vi "dataCube.vi"(10 "Enum":enum16{"clear", "read", "write"}(ring)=enum."write", 11 "imageCube":i32[][][](array[numeric])) -> (1 "imageCubeBkgSubstractedRefDivided":i32[][][](array[numeric]), 2 "imageCubeBkgSubstracted":i32[][][](array[numeric]), 3 "imageCubeOut":i32[][][](array[numeric]))   [LabVIEW 2016]
uses:
  imageSettings.vi
panel:
  out "ref":i32[][](graph)
  out "bkg":i32[][](graph)
  out "raw":i32[][](graph)
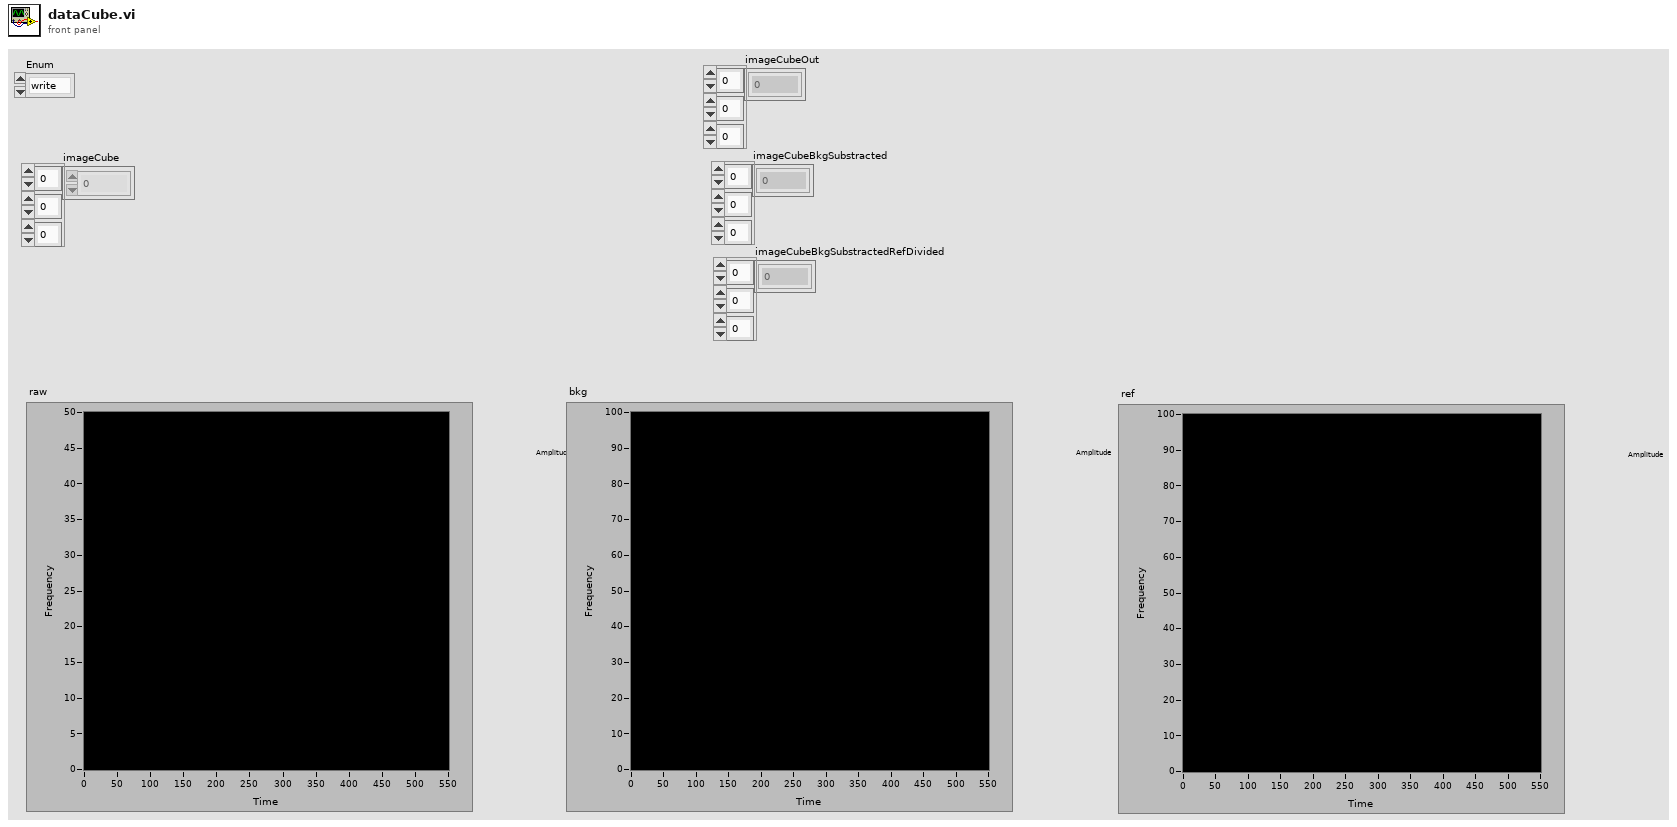
[diagram p1: front panel]
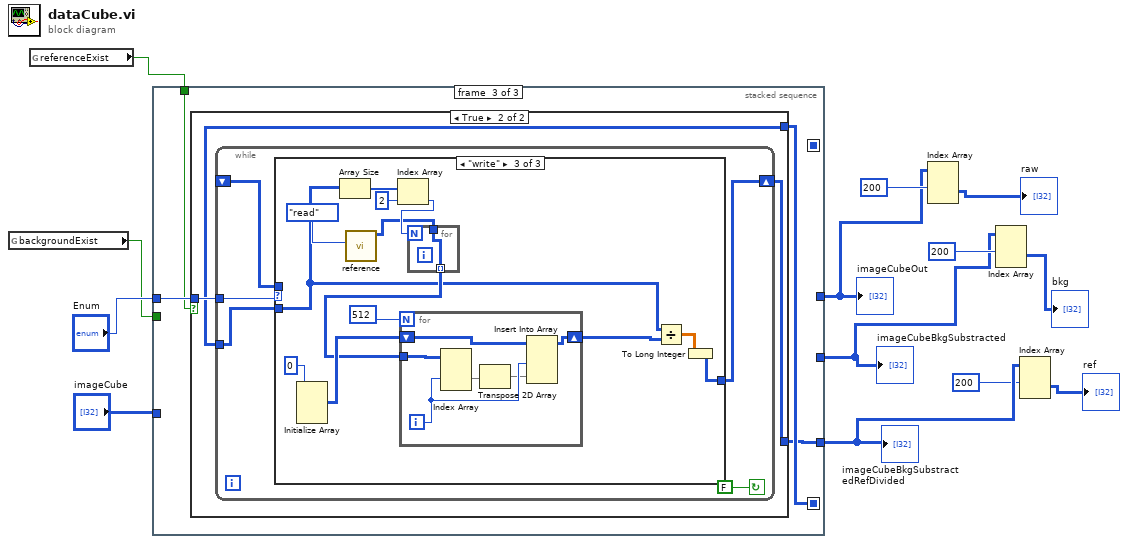
[diagram p0: block diagram]
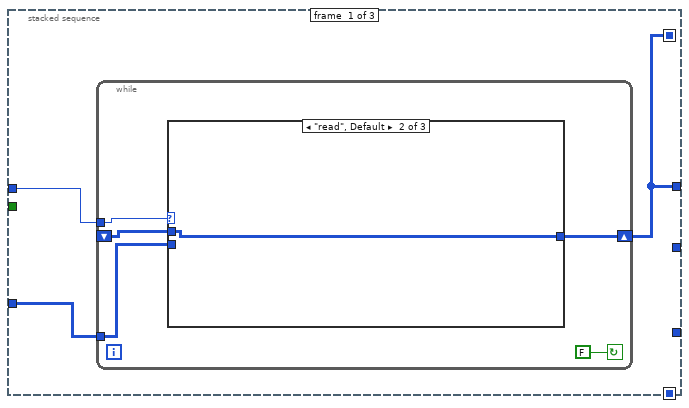
[diagram p2: hidden frame]
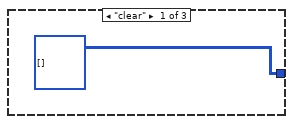
[diagram p3: hidden frame]
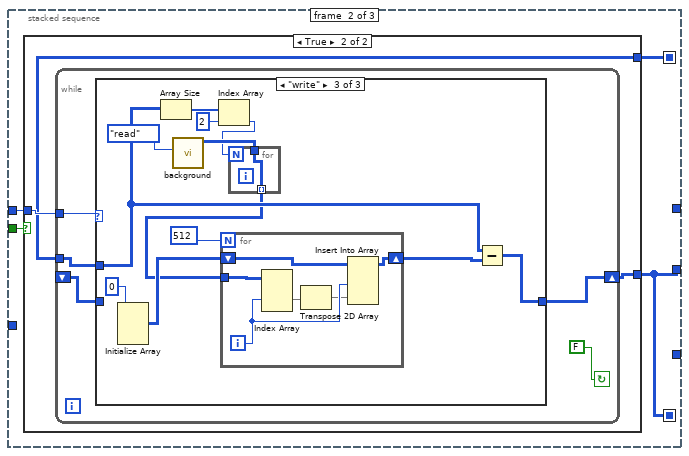
[diagram p5: hidden frame]
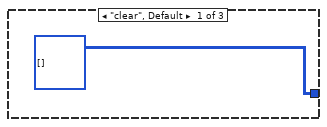
[diagram p7: hidden frame]
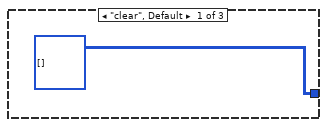
[diagram p10: hidden frame]
diagram:
  n1 = global read "imageSettings.vi" "backgroundExist"() -> (w10:bool)
  n2 = global read "imageSettings.vi" "referenceExist"() -> (w11:bool)
  n3 = stacked-sequence {
    seq-local: [w14 _ _] -> [_ w28 _]
    seq-local: [_ w27 _] -> [_ _ w61]
    tunnel: "Enum" -> [w16 w26 w59]
    tunnel: [w14 _ _] -> w2
    tunnel: "imageCube" -> [w15 _ _]
    tunnel: [_ w27 _] -> w5
    tunnel: [_ _ w60] -> w9
    tunnel: w11 -> [_ _ w58]
    tunnel: w10 -> [_ w25 _]
    frame #0 {
      n4 = while {
        tunnel: w16 -> [w20]
        shift-right: [w19] -> w14
        shift-left: _ -> [w17]
        tunnel: w15 -> [w18]
        stop <- FALSE continue-if-true
        n5 = case shown="\"read\", Default" w20 {
          tunnel: w18 -> [_ _ w24]
          tunnel: [i32[][][] [] ("imageCube") w23 w24] -> w19
          tunnel: w17 -> [_ w23 _]
          frame "clear" {
          }
          frame "read", Default {
          }
          frame "write" {
          }
        }
      }
    }
    frame #1 {
      n6 = case shown="True" w25 {
        tunnel: w28 -> [_ w29]
        tunnel: [_ w31] -> w27
        tunnel: w26 -> [_ w30]
        frame False {
        }
        frame True {
          n7 = while {
            shift-right: [w36] -> w31
            shift-left: _ -> [w32]
            tunnel: w30 -> [w34]
            tunnel: w29 -> [w33]
            stop <- FALSE continue-if-true
            n8 = case shown="\"write\"" w34 {
              tunnel: w33 -> [_ _ w50]
              tunnel: [i32[][][] [] ("imageCube") w38 w45] -> w36
              tunnel: w32 -> [_ w38 _]
              frame "clear", Default {
              }
              frame "read" {
              }
              frame "write" {
                n9 = Initialize Array(0) -> (w43:i32[][][])  [unwired: 3 in]
                n10 = Array Size(array=w50) -> (size(s)=w49:i32[])
                n11 = call "background.vi"("Enum"=enum16{"clear", "read", "write"}."read") -> ("backgroundImageOut"=w46:i32[][])  [unwired: 10 in]
                n12 = Index Array(array=w49, index=2) -> (element=w44:i32)
                n13 = for {
                  N: w44 -> [_]
                  tunnel: w46 -> [w57]
                  tunnel: [w57] -> w41 mode=indexing
                }
                n14 = for {
                  N: 512 -> [_]
                  tunnel: w41 -> [w56]
                  shift-right: [w54] -> w39
                  shift-left: w43 -> [w53]
                  i -> [w52]
                  n15 = Index Array(array=w56, index (dim 1)=w52) -> (element=w55:i32[][])  [unwired: 2 in]
                  n16 = Transpose 2D Array(2D array=w55) -> (transposed array=w51:i32[][])
                  n17 = Insert Into Array(array=w53, index (dim 1)=w52, new element=w51) -> (w54:i32[][][])  [unwired: 2 in]
                }
                n18 = Subtract(x=w50, y=w39) -> (x-y=w45:i32[][][])
              }
            }
          }
        }
      }
    }
    frame #2 {
      n19 = case shown="True" w58 {
        tunnel: w61 -> [_ w62]
        tunnel: [_ w64] -> w60
        tunnel: w59 -> [_ w63]
        frame False {
        }
        frame True {
          n20 = while {
            shift-right: [w68] -> w64
            shift-left: _ -> [w66]
            tunnel: w63 -> [w67]
            tunnel: w62 -> [w65]
            stop <- FALSE continue-if-true
            n21 = case shown="\"write\"" w67 {
              tunnel: w66 -> [_ w71 _]
              tunnel: [i32[][][] [] ("imageCube") w71 w73] -> w68
              tunnel: w65 -> [_ _ w72]
              frame "clear", Default {
              }
              frame "read" {
              }
              frame "write" {
                n22 = Initialize Array(0) -> (w80:i32[][][])  [unwired: 3 in]
                n23 = Array Size(array=w72) -> (size(s)=w84:i32[])
                n24 = call "reference.vi"("Enum"=enum16{"clear", "read", "write"}."read") -> ("referenceImageOut"=w74:i32[][])  [unwired: 10 in]
                n25 = Index Array(array=w84, index=2) -> (element=w81:i32)
                n26 = for {
                  N: w81 -> [_]
                  tunnel: w74 -> [w91]
                  tunnel: [w91] -> w78 mode=indexing
                }
                n27 = for {
                  N: 512 -> [_]
                  tunnel: w78 -> [w90]
                  shift-right: [w88] -> w76
                  shift-left: w80 -> [w87]
                  i -> [w86]
                  n28 = Index Array(array=w90, index (dim 1)=w86) -> (element=w89:i32[][])  [unwired: 2 in]
                  n29 = Transpose 2D Array(2D array=w89) -> (transposed array=w85:i32[][])
                  n30 = Insert Into Array(array=w87, index (dim 1)=w86, new element=w85) -> (w88:i32[][][])  [unwired: 2 in]
                }
                n31 = Divide(x=w72, y=w76) -> (x/y=w82:dbl[][][])
                n32 = To Long Integer(number=w82) -> (32bit integer=w73:i32[][][])
              }
            }
          }
        }
      }
    }
  }
  "imageCubeOut" <- w2
  "imageCubeBkgSubstracted" <- w5
  "imageCubeBkgSubstractedRefDivided" <- w9
  n33 = Index Array(array=w2, index (dim 0)=200 ("index (page)")) -> (element=→"raw":i32[][])  [unwired: 2 in]
  n34 = Index Array(array=w5, index (dim 0)=200 ("index (page)")) -> (element=→"bkg":i32[][])  [unwired: 2 in]
  n35 = Index Array(array=w9, index (dim 0)=200 ("index (page)")) -> (element=→"ref":i32[][])  [unwired: 2 in]
